vi "runDO_tt.vi"   [LabVIEW 2013]
types:
  T1 = typedef "LVRectTypeDef.ctl" = cluster{"Left":i16, "Top":i16, "Right":i16, "Bottom":i16}
  T2 = cluster{"Xpixels":i32, "Vxminref":dbl, "Vxmaxref":dbl, "P":dbl, "Ypixels":i32, "Vyminref":dbl, "Vymaxref":dbl, "srate":sgl, "sAOxy":i32, "timeout":dbl, "type":string, "date":string, "time":string, "Colormap":u16, "Drawing Mode":u16, "Scanning Mode":u16, "square pixels":bool, "square matrix":bool, "Xpixels Img":i32, "Vx-min Img":dbl, "VX-max Img":dbl, "Ypixels Img":i32, "Vy-min Img":dbl, "Vy-max Img ":dbl, "Angle Img":dbl, "autoshutter":bool, "finite":bool, "cont":bool, "wavdet":bool, "measpoints":i32, "avpp":i32, "bufferAO":i32, "bufferAI":i32, "starttick":u32, "waveform":path, "Vx-ref":dbl, "Vy-ref":dbl, "refreshrate":dbl, "refreshbuffer":i32, "tt_cycles":i32, "motorref":refnum<k7>, "mirrorswitch":refnum<k7>, "sample mode":i32, "maxbufferAI":i32, "sampletreshold":dbl, "srateAODO":sgl, "bin":sgl, "Pel":sgl, "Angle draw":dbl, "srate Img":sgl, "ROIimg_plotbounds":T1, "auto OD":bool, "ODfilt":u16, "reset AO_DO":bool, "aAI":i32[], "aCI":i32[], "aAO":i32[], "aDO":i32[]}
  T3 = cluster{"Min Voltage sq (mV)":dbl, "Max voltage sq (mV)":dbl, "Duty cycle sq(%)":dbl, "Voltage freq. sq(Hz)":dbl, "# cycles sq":u32, "meastype":enum16{"sealtest hekcells", "sealtest neurons", "Manual", "from file"}, "sample rate":dbl, "amp":dbl, "sample mode":i32, "refreshbuffer":i32, "timeout":sgl, "Min Voltage tri (mV)":dbl, "Max voltage tri (mV)":dbl, "Voltage freq. tri(Hz)":dbl, "# cycles tri":u32, "Voltage step ":bool, "Voltage triangle":bool, "file":bool, "refreshrate":dbl, "sAOXY":dbl, "avpp":i32, "Pel":dbl, "bin":dbl, "lAO":i32[], "lDO":i32[]}
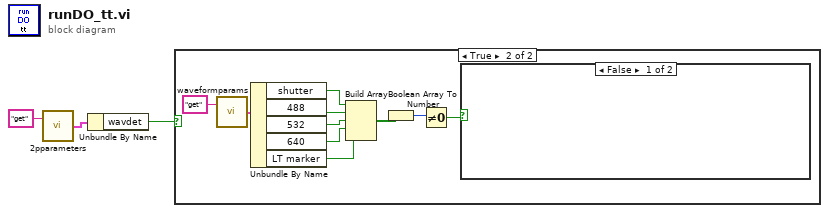
[diagram p0: block diagram]
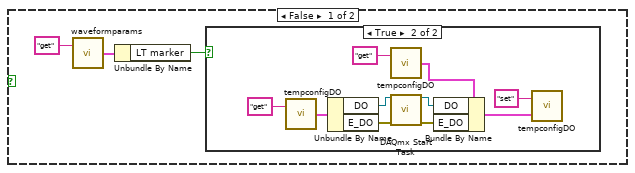
[diagram p2: hidden frame]
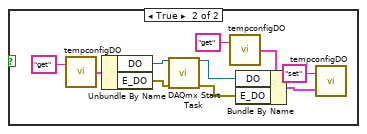
[diagram p4: hidden frame]
diagram:
  n1 = call "2pparameters.vi"("command"="get") -> ("params out"=w2:T2)  [unwired: 1 in]
  n2 = Unbundle By Name(w2) -> ("wavdet"=w1:bool)
  n3 = case shown="True" w1 {
    frame False {
      n4 = call "waveformparams.vi"("command"="get") -> ("Params out"=w5:T3)  [unwired: 1 in]
      n5 = Unbundle By Name(w5) -> ("LT marker"=w6:bool)
      n6 = case shown="True" w6 {
        frame False {
        }
        frame True {
          n7 = call "tempconfigDO.vi"("command"="get") -> ("Temp Config out"=w13:cluster{"DO":refnum<k21>, "E_DO":errorcluster})  [unwired: 1 in]
          n8 = Unbundle By Name(w13) -> ("DO"=w12:refnum<k21>, "E_DO"=w11:errorcluster)
          n9 = call "tempconfigDO.vi"("command"="get") -> ("Temp Config out"=w10:cluster{"DO":refnum<k21>, "E_DO":errorcluster})  [unwired: 1 in]
          n10 = call <vilib>:"DAQmx Start Task.vi"("task/channels in"=w12, "error in"=w11) -> ("task out"=w9:refnum<k21>, "error out"=w8:errorcluster)  [unwired: 12 in]
          n11 = Bundle By Name(cluster=w10, "DO"=w9, "E_DO"=w8) -> (w7:cluster{"DO":refnum<k21>, "E_DO":errorcluster})
          n12 = call "tempconfigDO.vi"("Temp Config in"=w7, "command"="set") -> ()  [unwired: 1 out]
        }
      }
    }
    frame True {
      n13 = call "waveformparams.vi"("command"="get") -> ("Params out"=w25:T3)  [unwired: 1 in]
      n14 = Unbundle By Name(w25) -> ("shutter"=w24:bool, "488"=w23:bool, "532"=w22:bool, "640"=w21:bool, "LT marker"=w17:bool)
      n15 = Build Array(w24, w23, w22, w21, w17) -> (w20:bool[])
      n16 = Boolean Array To Number(Boolean array=w20) -> (number=w19:u32)
      n17 = Not Equal To 0?(x=w19) -> (x != 0?=w18:bool)
      n18 = case shown="False" w18 {
        frame False {
        }
        frame True {
          n19 = call "tempconfigDO.vi"("command"="get") -> ("Temp Config out"=w33:cluster{"DO":refnum<k21>, "E_DO":errorcluster})  [unwired: 1 in]
          n20 = Unbundle By Name(w33) -> ("DO"=w32:refnum<k21>, "E_DO"=w31:errorcluster)
          n21 = call <vilib>:"DAQmx Start Task.vi"("task/channels in"=w32, "error in"=w31) -> ("task out"=w29:refnum<k21>, "error out"=w28:errorcluster)  [unwired: 12 in]
          n22 = call "tempconfigDO.vi"("command"="get") -> ("Temp Config out"=w30:cluster{"DO":refnum<k21>, "E_DO":errorcluster})  [unwired: 1 in]
          n23 = Bundle By Name(cluster=w30, "DO"=w29, "E_DO"=w28) -> (w27:cluster{"DO":refnum<k21>, "E_DO":errorcluster})
          n24 = call "tempconfigDO.vi"("Temp Config in"=w27, "command"="set") -> ()  [unwired: 1 out]
        }
      }
    }
  }
